vi "Write TOML File (LV).vi"(8 "error in (no error)":errorcluster, 10 "Value":variant, 11 "file path (use dialog)":path) -> (0 "error out":errorcluster)   [LabVIEW 2017, in "TOML.lvlib"]
uses:
  TOML.lvlib
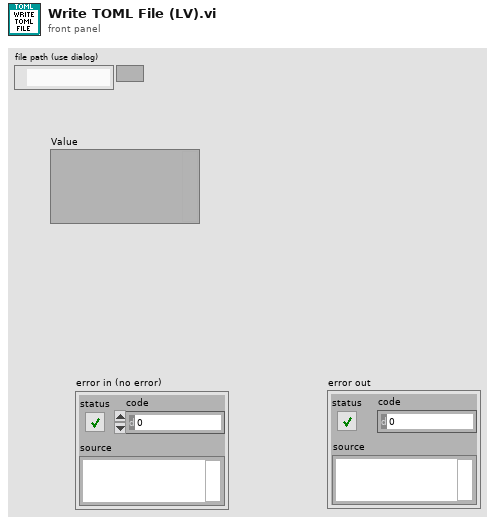
[diagram p1: front panel]
types:
  T1 = enum16{"open", "replace", "create", "open or create", "replace or create", "replace or create with confirmation"}
  T2 = typedef "TOML.lvlib/TOML Value.ctl" = cluster{"\\type":enum16{"Table", "Array", "String", "Integer", "Float", "Boolean", "Offset Date-Time", "Local Date-Time", "Local Date", "Local Time"}, "ÿýÿýÿýÿýÿýÿþÿýÿýÿý%LV-TOML.lvlib:TOML Key-Value Pair.ctlÿýÿýÿýÿýÿýÿþÿýÿýÿýLV-TOML.lvlib:TOML Value.ctl$":variant}
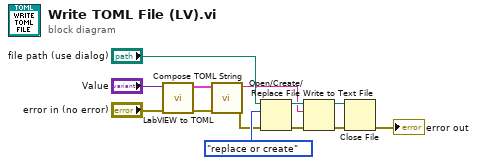
[diagram p0: block diagram]
diagram:
  n1 = call "LabVIEW to TOML.vi"("error in (no error)"="error in (no error)", "LV Value"="Value") -> ("error out"=w2:errorcluster, "TOML Value"=w4:T2)  [unwired: 8 in]
  n2 = call "Compose TOML String.vi"("error in (no error)"=w2, "Value"=w4) -> ("error out"=w1:errorcluster, "String"=w3:string)  [unwired: 8 in]
  n3 = Open/Create/Replace File(file path (use dialog)="file path (use dialog)", error in=w1, operation (0:open)=T1."replace or create") -> (refnum out=w9:refnum<file>, error out=w10:errorcluster)  [unwired: 3 in, 1 out]
  n4 = Write to Text File(file (use dialog)=w9, text=w3, error in=w10) -> (refnum out=w7:refnum<file>, error out=w8:errorcluster)  [unwired: 1 in, 1 out]
  n5 = Close File(refnum=w7, error in=w8) -> (error out=→"error out":errorcluster)  [unwired: 1 out]
